vi "S&E Base String.vi"(5 "Delimiter(;)":string=";", 7 "E&S Message":T2, 9 "error in (no error)":errorcluster, 12 "Time format(%T)":string="%T") -> (1 "date/time string":string, 2 "Location/ID":string, 3 "Elevated priority":bool, 6 "Measage text file Header string":string, 8 "Message content":variant, 10 "error out":errorcluster, 13 "Sub ID":u16, 14 "Type":T1)   [LabVIEW 2011]
uses:
  emi Lib/System 01/0 - General/S&E reporting/Private/_emi_ S&E Message.ctl
  emi Lib/System 01/0 - General/S&E reporting/Private/_emi_ S&E Message type.ctl
  Application Structure/System ID.ctl
  Application Structure/Loop ID.ctl
  <vilib>/Utility/VariantDataType/VariantType.lvlib
panel:
  in  "Loop Type":variant
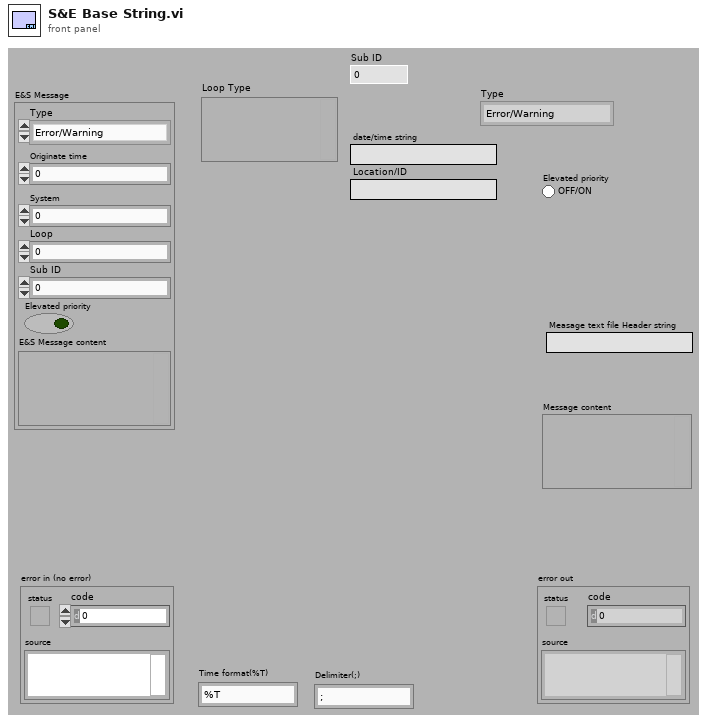
[diagram p1: front panel]
types:
  T1 = typedef "_emi_ S&E Message type.ctl" = enum16{"Error/Warning", "Note", "Debug", "Event", "Alarm Analog", "Alarm Digital", "Annotation"}
  T2 = typedef "_emi_ S&E Message.ctl" = cluster{"Type":T1, "Originate time":dbl, "System":u8, "Loop":u16, "Sub ID":u16, "Elevated priority":bool, "E&S Message content":variant}
  T3 = typedef "Loop ID.ctl" = enum16{"Main-QSM", "Main-Dialog", "Main-Ind Upd", "Main-Graph Upd", "Main-Debug", "Main-DebugW1", "Main-DebugW2", "Main-SE Handler", "Interface-PCP", "Interface-CANbus", "Interface-Modem", "Var Handling-Beat", "Var Handling-From PCP", "Var Handling-File storage", "Var Handling-From Tool", "GUI-GrphW Mast", "GUI-GrphW Slav", "SIM-Tool W1", "SIM-Tool W2", "Alm-Sound", "LEIN-motor", "Tool data gatherer Qer", "Tool Data LEIN STAT2 dekoder", "Indicator Value Update", "Tool STAT2 dedicated reader", "Tool ID handler", "Detail View L1", "Detail View L2", "Main display enable view", "Sequence runner", "Voltage setpoint", "Resistance setpoint", "Stroker Wizard L1", "Stroker Wizard L2", "Alarm Handling"}
  T4 = typedef "System ID.ctl" = enum16{"Host"}
  T5 = typedef "VariantType.lvlib/Type.ctl" = enum8{"Invalid Type", "Void", "I8", "I16", "I32", "I64", "U8", "U16", "U32", "U64", "Single Float", "Double Float", "Extended Float", "Single Complex", "Double Complex", "Extended Complex", "Enum U8", "Enum U16", "Enum U32", "Enum U64", "Single Float With Unit", "Double Float With Unit", "Extended Float With Unit", "Single Complex with Unit", "Double Complex with Unit", "Extended Complex with Unit", "Boolean", "String", "Path", "Picture", "Tag", "Array", "Cluster", "Variant", "LV Variant", "Waveform", "Timestamp", "Digital Waveform", "Digital Data", "ExpressData", "Refnum", "External Data", "VI", "Poly VI", "LabVIEW Class Instance", "Fixed Point"}
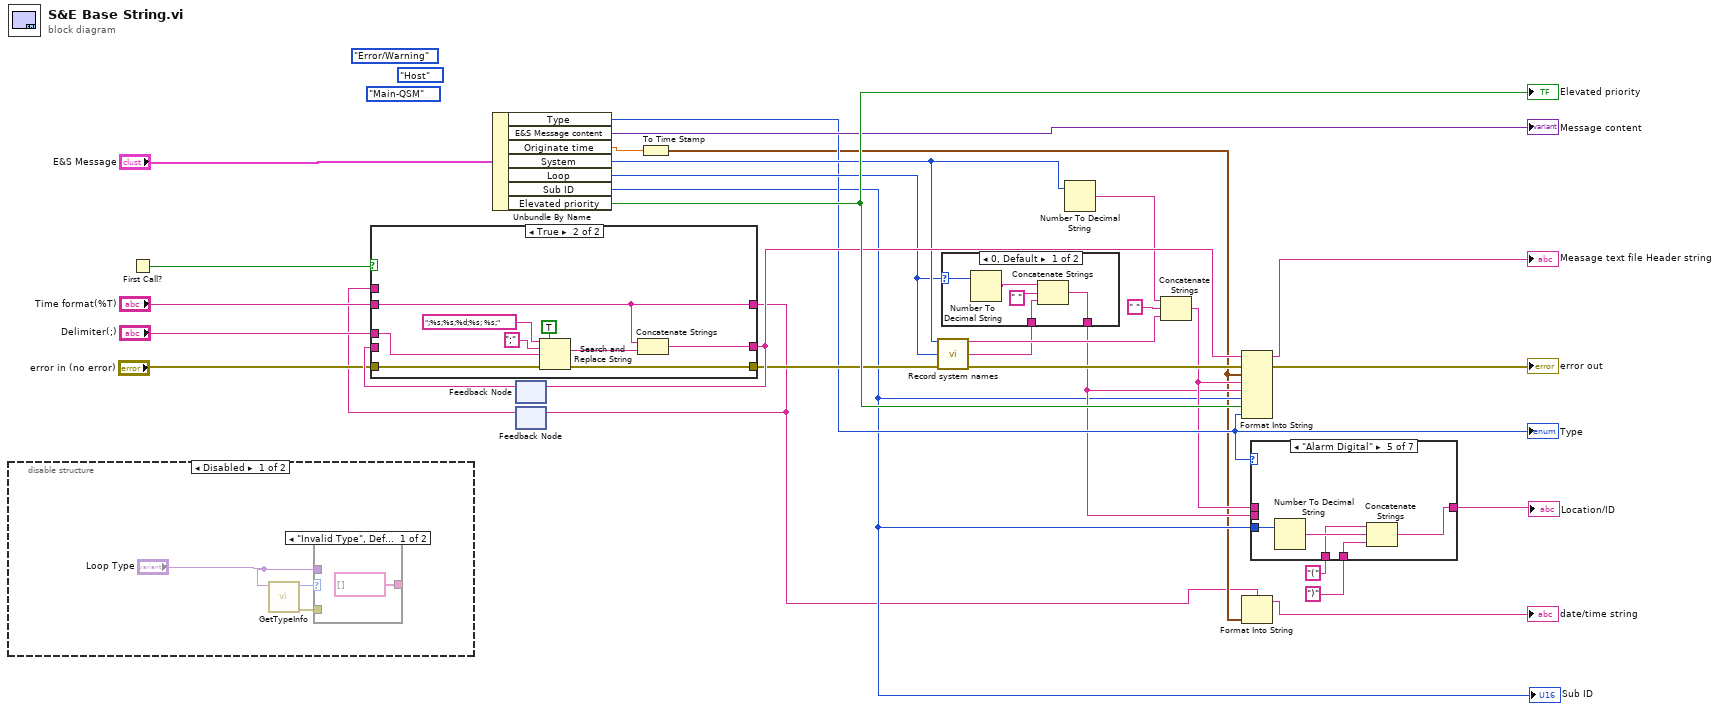
[diagram p0: block diagram]
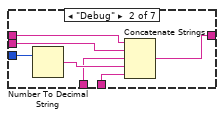
[diagram p3: hidden frame]
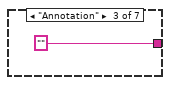
[diagram p4: hidden frame]
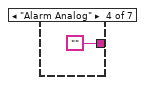
[diagram p5: hidden frame]
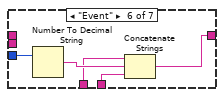
[diagram p6: hidden frame]
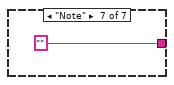
[diagram p7: hidden frame]
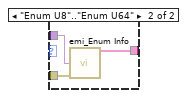
[diagram p9: hidden frame]
diagram:
  (unwired) _emi__S&E_Message_type."Error/Warning" ("Type")
  (unwired) Loop_ID."Main-QSM" ("Loop ID")
  (unwired) System_ID."Host" ("Loop ID")
  n1 = disable-structure shown="Disabled" {
    frame Disabled {
      n2 = call <vilib>:"GetTypeInfo.vi"("Variant"="Loop Type") -> ("error out"=w33:errorcluster, "Type Enum"=w34:T5)  [unwired: 6 in, 3 out]
      n3 = case shown="\"Invalid Type\", Default" w34 {
        tunnel: "Loop Type" -> [_ w38]
        tunnel: w33 -> [_ w37]
        tunnel: [string[] [] ("Text Elements") w36] -> _
        frame "Invalid Type", Default {
        }
        frame "Enum U8".."Enum U64" {
          n4 = call "emi_Enum Info.vi"("Enum"=w38, "error in (no error)"=w37) -> ("Text Elements"=w36:string[])  [unwired: 10 in, 3 out]
        }
      }
    }
    frame Enabled {
    }
  }
  n5 = First Call?() -> (First Call?: T/F=w29:bool)
  n6 = Unbundle By Name("E&S Message") -> ("Type"=w11:T1, "E&S Message content"=→"Message content":variant, "Originate time"=w24:dbl, "System"=w14:u8, "Loop"=w13:u16, "Sub ID"=w6:u16, "Elevated priority"=w31:bool)
  "Elevated priority" <- w31
  "Type" <- w11
  "Sub ID" <- w6
  n7 = feedback #1() -> (w30:string)  [unwired: 1 in]
  n8 = feedback #2() -> (w12:string)  [unwired: 1 in]
  n9 = case shown="True" w29 {
    tunnel: [w41 w50] -> w21
    tunnel: "Time format(%T)" -> [_ w42]
    tunnel: "Delimiter(;)" -> [_ w46]
    tunnel: w30 -> [w41 _]
    tunnel: [w40 w44] -> w17
    tunnel: "error in (no error)" -> [w40 w43]
    tunnel: [w39 w42] -> w2
    tunnel: w12 -> [w39 _]
    frame False {
    }
    frame True {
      n10 = Search and Replace String(replace all?=TRUE ("replace all? (F)"), input string=";%s;%s;%d;%s; %s;" ("format string"), search string=";", replace string=w46, error in=w43) -> (result string=w49:string, error out=w44:errorcluster)  [unwired: 3 in, 2 out]
      n11 = Concatenate Strings(w42, w49) -> (w50:string)
    }
  }
  n12 = feedback-in #1(w21) -> ()
  n13 = feedback-in #2(w2) -> ()
  n14 = To Time Stamp(1:w24) -> (0:w3:timestamp)
  n15 = call "Record system names.vi"("System(0)"=w14, "Loop(0)"=w13, "error in (no error)"=w17) -> ("System navn"=w15:string, "Loop name"=w9:string, "error out"=w16:errorcluster)  [unwired: 8 in, 2 out]
  n16 = case shown="0, Default" w13 {
    selector: w13 -> [w51 _]
    tunnel: [w53 w56] -> w7
    tunnel: w9 -> [w52 w56]
    frame 0, Default {
      n17 = Number To Decimal String(number=w51) -> (decimal integer string=w55:string)  [unwired: 1 in]
      n18 = Concatenate Strings(w55, " " ("string"), w52) -> (w53:string)
    }
    frame 9999 {
    }
  }
  n19 = Number To Decimal String(number=w14) -> (decimal integer string=w19:string)  [unwired: 1 in]
  n20 = Concatenate Strings(w19, " " ("string"), w15) -> (w8:string)
  n21 = Format Into String(format string=w21, error in=w16, w3, w8, w7, w6, w31, w11) -> (resulting string=→"Measage text file Header string":string, error out=→"error out":errorcluster)  [unwired: 1 in]
  n22 = Format Into String(format string=w2, w3) -> (resulting string=→"date/time string":string)  [unwired: 2 in, 1 out]
  n23 = case shown="\"Alarm Digital\"" w11 {
    tunnel: [w57 w58 "" ("date/time string") "" w67 w72 "" ("date/time string")] -> w10
    tunnel: w8 -> [w57 w62 _ _ _ _ _]
    tunnel: w7 -> [_ w61 _ _ _ _ _]
    tunnel: w6 -> [_ w64 _ _ w71 w76 _]
    tunnel: "(" ("string") -> [_ w60 _ _ w69 w74 _]
    tunnel: ")" ("string") -> [_ w59 _ _ w68 w73 _]
    frame "Error/Warning", Default {
    }
    frame "Debug" {
      n24 = Number To Decimal String(number=w64) -> (decimal integer string=w63:string)  [unwired: 1 in]
      n25 = Concatenate Strings(w62, w61, w60, w63, w59) -> (w58:string)
    }
    frame "Annotation" {
    }
    frame "Alarm Analog" {
    }
    frame "Alarm Digital" {
      n26 = Number To Decimal String(number=w71) -> (decimal integer string=w70:string)  [unwired: 1 in]
      n27 = Concatenate Strings(w69, w70, w68) -> (w67:string)
    }
    frame "Event" {
      n28 = Number To Decimal String(number=w76) -> (decimal integer string=w75:string)  [unwired: 1 in]
      n29 = Concatenate Strings(w74, w75, w73) -> (w72:string)
    }
    frame "Note" {
    }
  }
  "Location/ID" <- w10
